vi "ControlFiAssaig.vi"(6 "Actiu":bool, 7 "PercentatgeCaiguda":dbl, 8 "FonsEscalaCaptador":dbl, 9 "ControlaCaigudaEntrada":bool, 10 "ValorActual":dbl, 11 "ValorMaxim":dbl) -> (1 "ControlaCaigudaSortida":bool, 2 "ParoRotura":bool, 3 "NouMaxim":dbl)   [LabVIEW 2017]
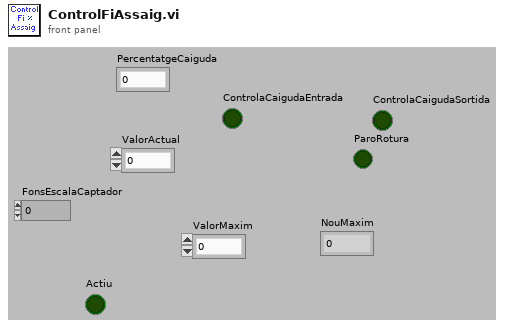
[diagram p1: front panel]
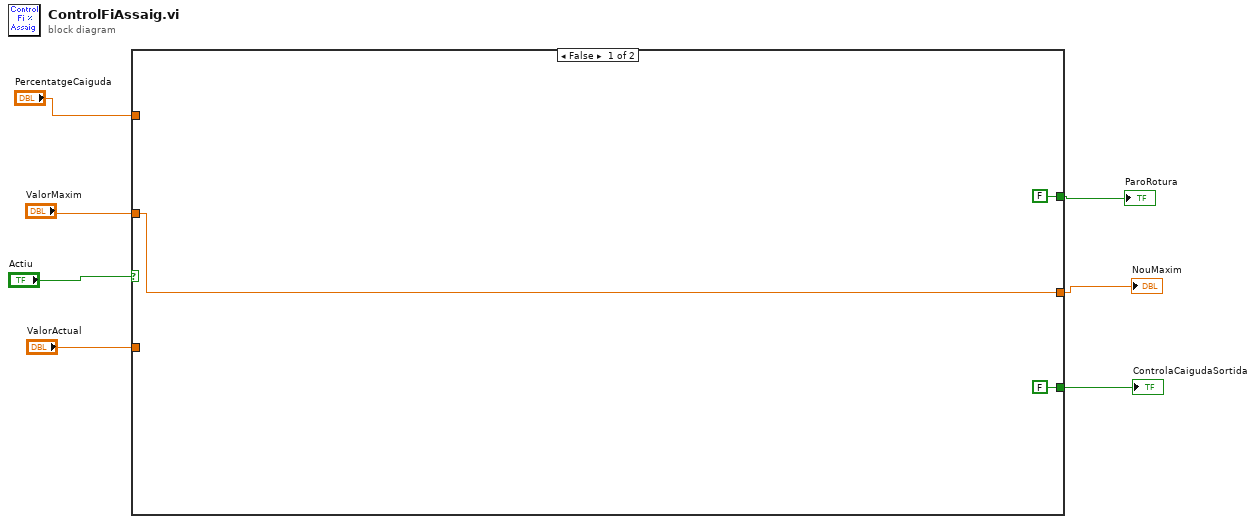
[diagram p0: block diagram]
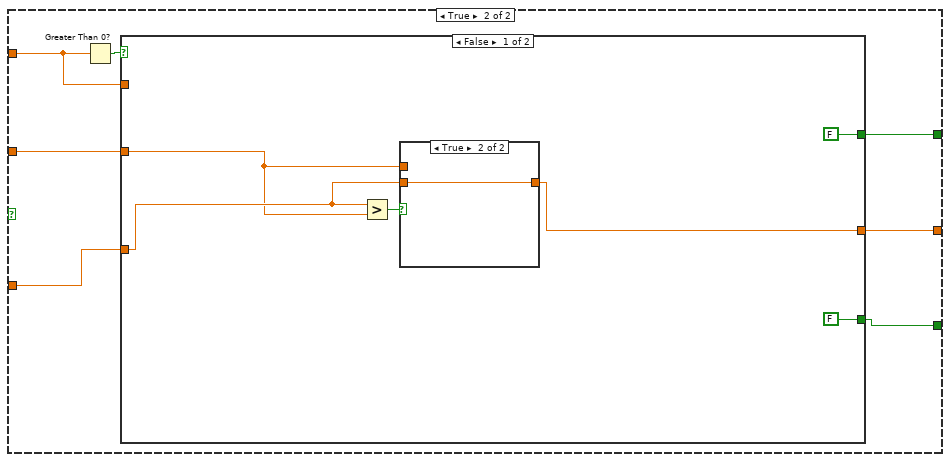
[diagram p2: hidden frame]
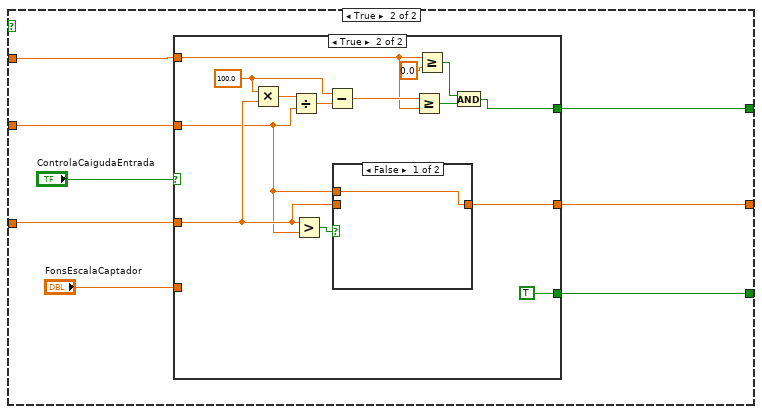
[diagram p4: hidden frame]
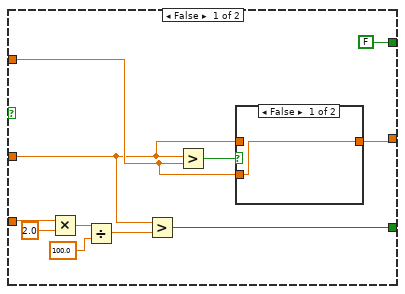
[diagram p5: hidden frame]
diagram:
  n1 = case shown="False" "Actiu" {
    tunnel: [FALSE w16] -> w7
    tunnel: [FALSE w15] -> w6
    tunnel: [w10 w14] -> w5
    tunnel: "PercentatgeCaiguda" -> [_ w13]
    tunnel: "ValorMaxim" -> [w10 w12]
    tunnel: "ValorActual" -> [_ w11]
    frame False {
    }
    frame True {
      n2 = Greater Than 0?(x=w13) -> (x > 0?=w17:bool)
      n3 = case shown="False" w17 {
        tunnel: w13 -> [_ w31]
        tunnel: [FALSE w30] -> w16
        tunnel: [FALSE w29] -> w15
        tunnel: w11 -> [w20 w28]
        tunnel: w12 -> [w18 w27]
        tunnel: [w19 w26] -> w14
        frame False {
          n4 = Greater?(x=w20, y=w18) -> (0:w21:bool)
          n5 = case shown="True" w21 {
            tunnel: w20 -> [_ w25]
            tunnel: [w24 w25] -> w19
            tunnel: w18 -> [w24 _]
            frame False {
            }
            frame True {
            }
          }
        }
        frame True {
          n6 = case shown="True" "ControlaCaigudaEntrada" {
            tunnel: [FALSE w47] -> w30
            tunnel: w28 -> [w36 w55]
            tunnel: w27 -> [w41 w53]
            tunnel: w31 -> [_ w49]
            tunnel: [w42 w54] -> w26
            tunnel: "FonsEscalaCaptador" -> [w40 _]
            tunnel: [w34 TRUE] -> w29
            frame False {
              n7 = Multiply(x=w40, y=2.0) -> (x*y=w38:dbl)
              n8 = Divide(x=w38, y=100.0) -> (x/y=w35:dbl)
              n9 = Greater?(x=w36, y=w35) -> (0:w34:bool)
              n10 = Greater?(x=w36, y=w41) -> (0:w43:bool)
              n11 = case shown="False" w43 {
                tunnel: w36 -> [_ w46]
                tunnel: [w45 w46] -> w42
                tunnel: w41 -> [w45 _]
                frame False {
                }
                frame True {
                }
              }
            }
            frame True {
              w56 = 100.0 ("x")
              n12 = Multiply(x=w56, y=w55) -> (x*y=w60:dbl)
              n13 = Divide(x=w60, y=w53) -> (x/y=w57:dbl)
              n14 = Greater?(x=w55, y=w53) -> (0:w59:bool)
              n15 = Subtract(x=w56, y=w57) -> (x-y=w58:dbl)
              n16 = case shown="False" w59 {
                tunnel: w55 -> [_ w62]
                tunnel: [w61 w62] -> w54
                tunnel: w53 -> [w61 _]
                frame False {
                }
                frame True {
                }
              }
              n17 = Greater Or Equal?(x=w58, y=w49) -> (x >= y?=w51:bool)
              n18 = Greater Or Equal?(x=w49, y=0.0) -> (x >= y?=w48:bool)
              n19 = And(x=w48, y=w51) -> (x .and. y?=w47:bool)
            }
          }
        }
      }
    }
  }
  "ParoRotura" <- w7
  "ControlaCaigudaSortida" <- w6
  "NouMaxim" <- w5
